vi "Append Port to Host String.vi"(0 "host in":string, 5 "port":u16) -> (4 "host out":string)   [LabVIEW 2009, in "AMC.lvlib"]
uses:
  AMC.lvlib
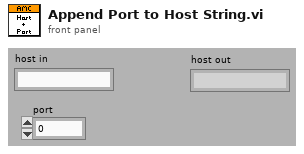
[diagram p1: front panel]
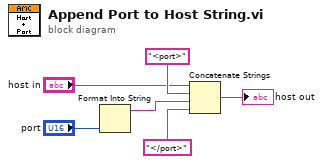
[diagram p0: block diagram]
diagram:
  n1 = Format Into String("port") -> (resulting string=w6:string)  [unwired: 3 in, 1 out]
  n2 = Concatenate Strings("host in", "<port>" ("string"), w6, "</port>" ("string")) -> (→"host out":string)
